vi "preregister_tools.vi"() -> ()   [LabVIEW 2018]
uses:
  controls/preregistration_data.ctl
panel:
  out "text":string
  in  "preregistration_data":T1 {"Starting serial number" format="%#_11g"}
  out "error out":errorcluster
  in  "close":bool
  out "Progress of preregistration data generation":u8(slide) scale=0.0..100.0
  out "Progress of mac_db.txt generation":u8(slide) scale=0.0..100.0
  in  "open":bool
  in  "run":bool
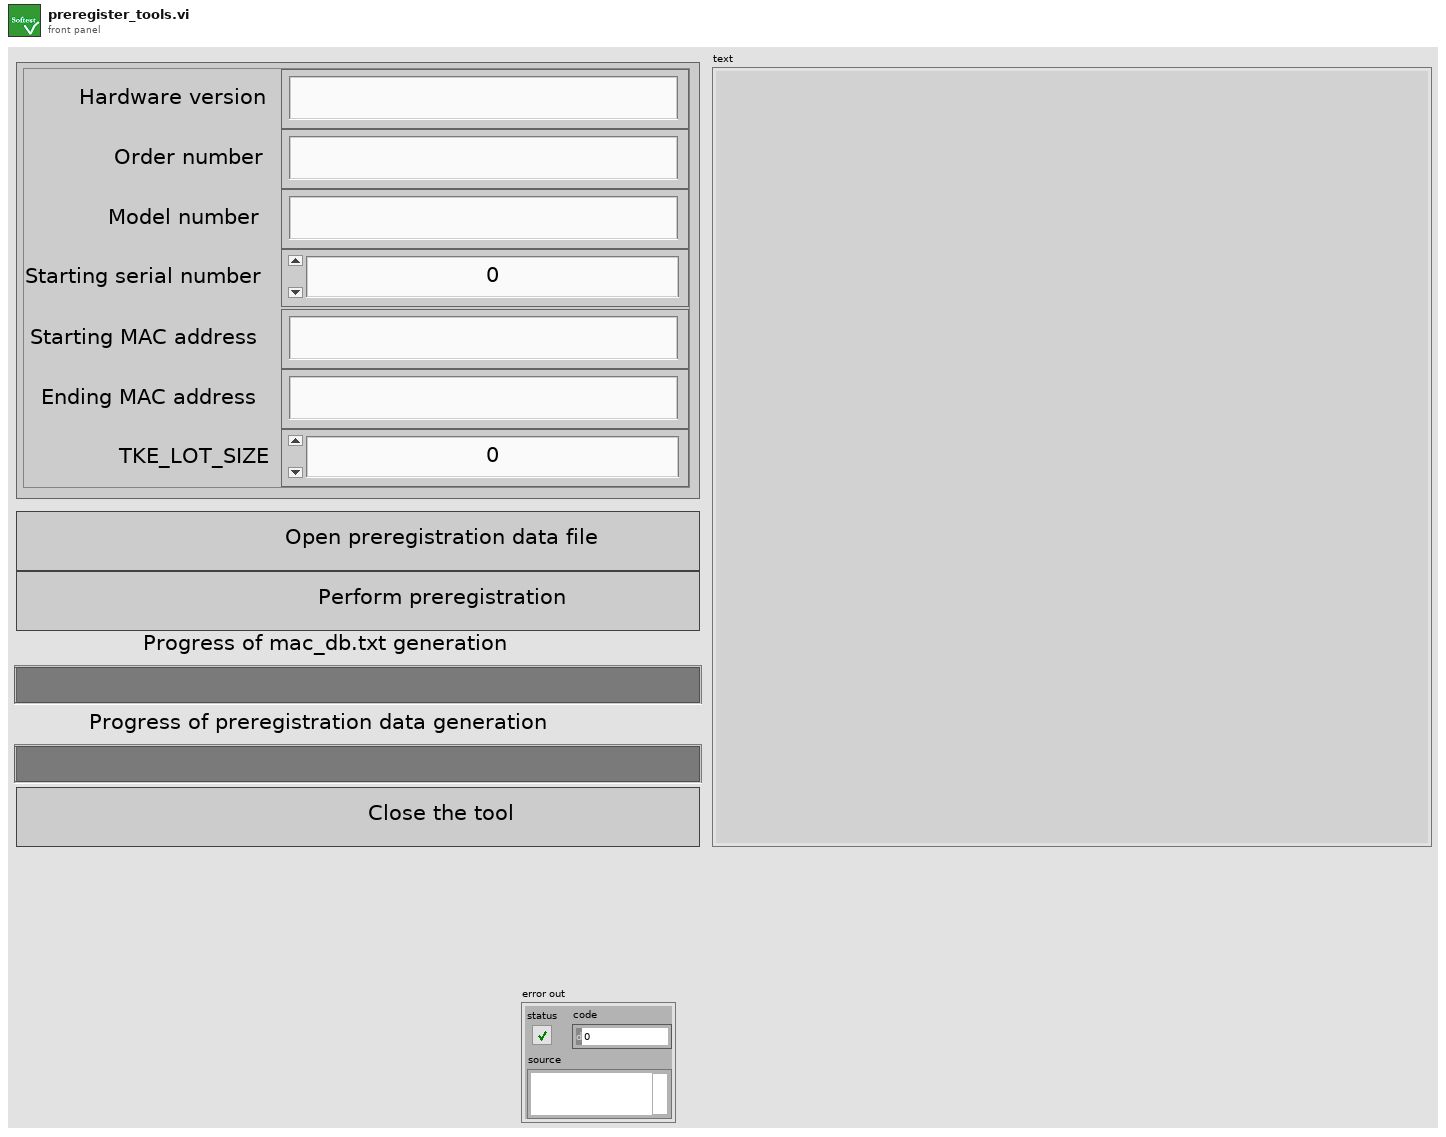
[diagram p1: front panel]
types:
  T1 = typedef "preregistration_data.ctl" = cluster{"Hardware version":string, "Order number":string, "Model number":string, "Starting serial number":i32, "Starting MAC address":string, "Ending MAC address":string, "TKE_LOT_SIZE":i32}
  T2 = enum32{"invalid app kind", "Development System", "Run Time System", "Student Edition", "Embedded LabVIEW", "Evaluation", "Custom"}
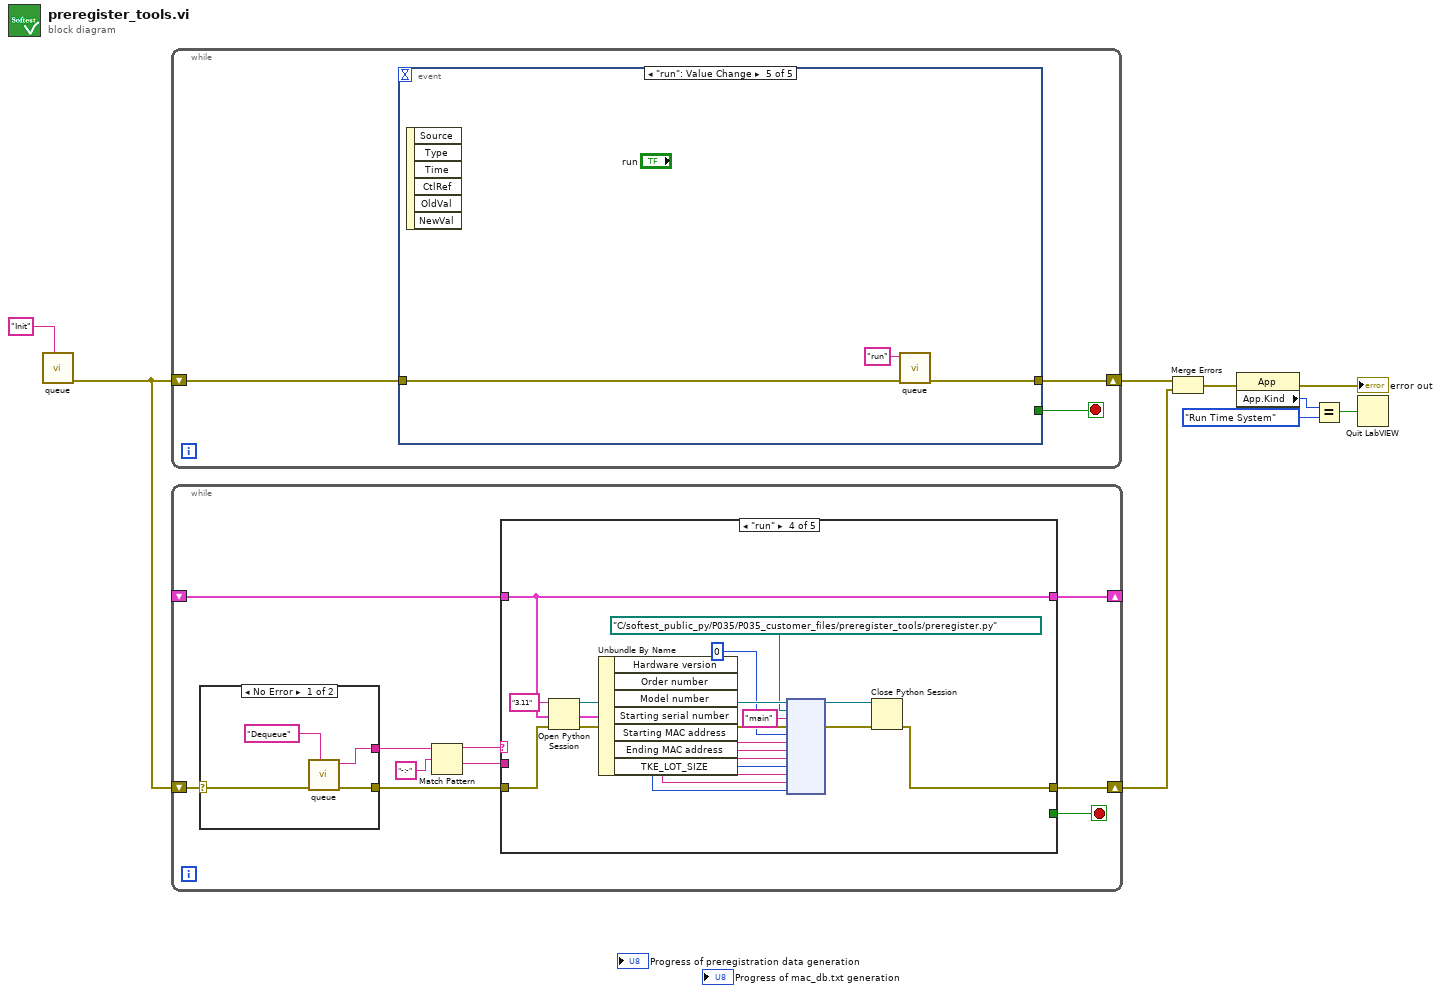
[diagram p0: block diagram]
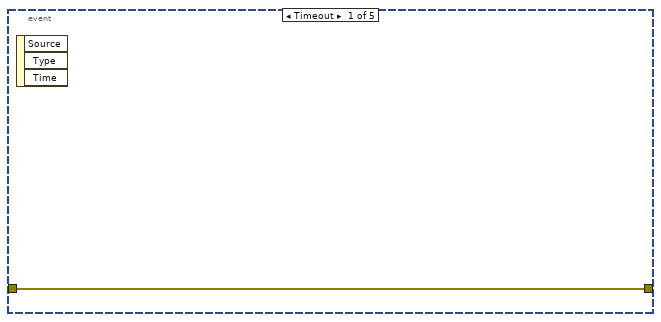
[diagram p2: hidden frame]
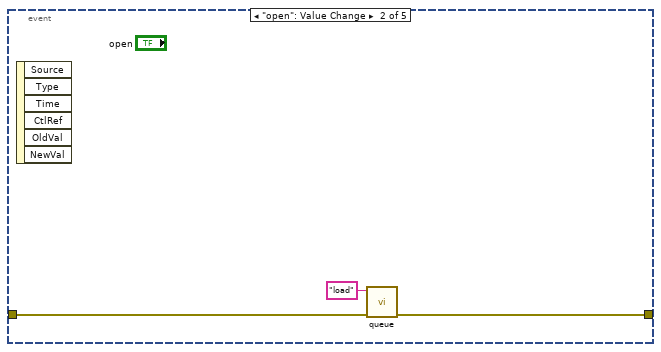
[diagram p3: hidden frame]
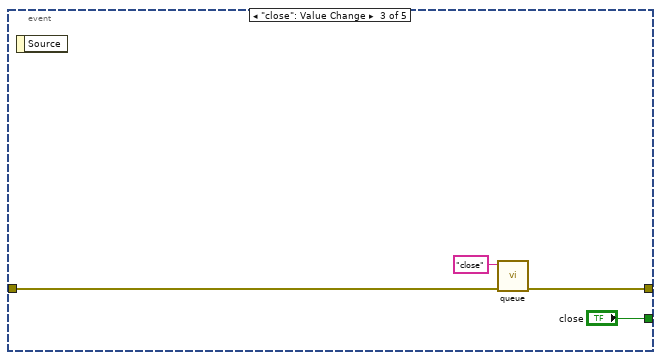
[diagram p4: hidden frame]
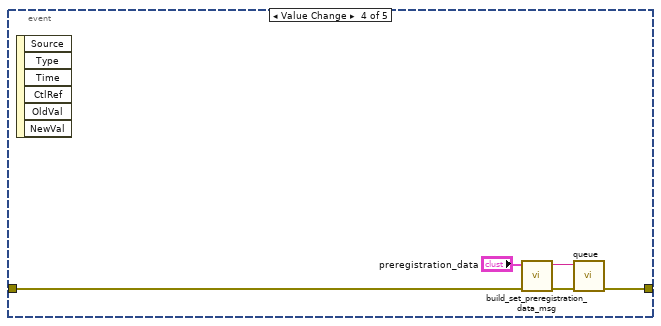
[diagram p5: hidden frame]
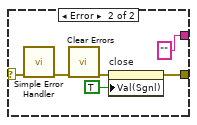
[diagram p6: hidden frame]
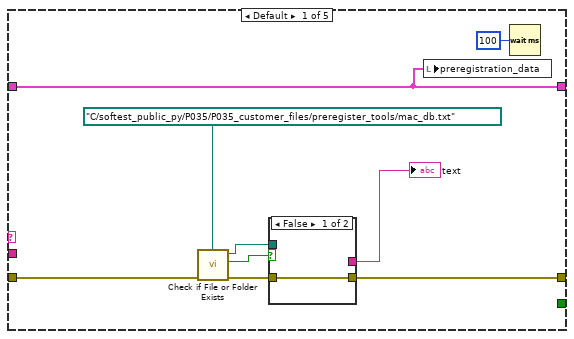
[diagram p7: hidden frame]
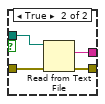
[diagram p8: hidden frame]
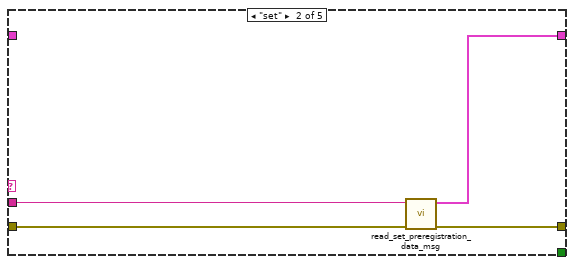
[diagram p9: hidden frame]
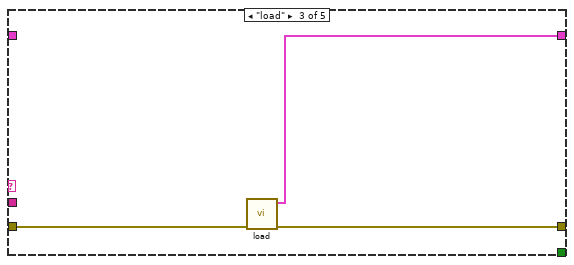
[diagram p10: hidden frame]
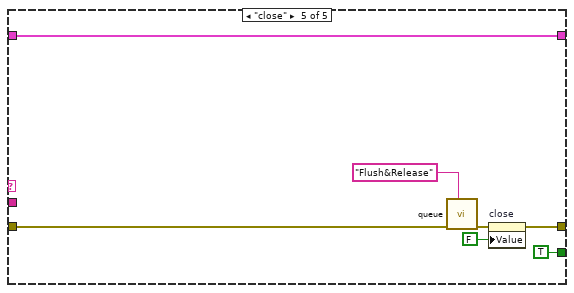
[diagram p11: hidden frame]
diagram:
  n1 = call "queue.vi"("action"="Init") -> ("error_out"=w8:errorcluster)  [unwired: 9 in, 1 out]
  n2 = while {
    shift-right: [w10] -> w7
    shift-left: w8 -> [w11]
    stop <- w12 stop-if-true
    n3 = event shown="[4] \"run\": Value Change" {
      selector: _ -> [_ _ _ _ _]
      dyn-events: _ -> [_ _ _ _ _]
      timeout: _ -> [_ _ _ _ _]
      tunnel: [_ _ "close" _ _] -> w12
      tunnel: w11 -> [w13 w16 w19 w24 w28]
      tunnel: [w13 w15 w18 w25 w27] -> w10
      event Timeout {
        n4 = event-data() -> ()  [unwired: 1 in, 3 out]
      }
      event "open": Value Change {
        n5 = event-data() -> ()  [unwired: 1 in, 6 out]
        n6 = call "queue.vi"("error_in"=w16, "element_in"="load") -> ("error_out"=w15:errorcluster)  [unwired: 8 in, 1 out]
      }
      event "close": Value Change {
        n7 = event-data() -> ()  [unwired: 1 in, 1 out]
        n8 = call "queue.vi"("error_in"=w19, "element_in"="close") -> ("error_out"=w18:errorcluster)  [unwired: 8 in, 1 out]
      }
      event Value Change {
        n9 = event-data() -> ()  [unwired: 1 in, 6 out]
        n10 = call "build_set_preregistration_data_msg.vi"("error_in"=w24, "preregistration_data"="preregistration_data") -> ("error_out"=w23:errorcluster, "command"=w22:string)  [unwired: 8 in]
        n11 = call "queue.vi"("error_in"=w23, "element_in"=w22) -> ("error_out"=w25:errorcluster)  [unwired: 8 in, 1 out]
      }
      event "run": Value Change {
        n12 = event-data() -> ()  [unwired: 1 in, 6 out]
        n13 = call "queue.vi"("error_in"=w28, "element_in"="run") -> ("error_out"=w27:errorcluster)  [unwired: 8 in, 1 out]
      }
    }
  }
  n14 = while {
    shift-right: [w37] -> w6
    shift-left: w8 -> [w35]
    shift-right: [w34] -> _
    shift-left: _ -> [w33]
    stop <- w38 stop-if-true
    n15 = case shown="No Error" w35 {
      selector: w35 -> [w39 w47]
      tunnel: [w42 w44] -> w36
      tunnel: [w41 "" ("element_out")] -> w32
      frame No Error {
        n16 = call "queue.vi"("action"="Dequeue", "error_in"=w39) -> ("error_out"=w42:errorcluster, "element_out"=w41:string)  [unwired: 8 in]
      }
      frame Error {
        n17 = call <vilib>:"Simple Error Handler.vi"("error in (no error)"=w47) -> ("error out"=w46:errorcluster)  [unwired: 4 in, 4 out]
        n18 = call <vilib>:"Clear Errors.vi"("error in (no error)"=w46) -> ("error out"=w45:errorcluster)  [unwired: 5 in, 1 out]
        n19 = property on="close" class="Bool (strict)"(error in=w45, "Val(Sgnl)"=TRUE) -> (error out=w44:errorcluster)  [unwired: 1 in, 1 out]
      }
    }
    n20 = Match Pattern(string=w32, regular expression="-:-") -> (before substring=w30:string, after substring=w29:string)  [unwired: 1 in, 2 out]
    n21 = case shown="\"run\"" w30 {
      tunnel: [_ _ _ _ TRUE] -> w38
      tunnel: w36 -> [w53 w66 w68 w82 w93]
      tunnel: [w54 w64 w69 w83 w90] -> w37
      tunnel: [w56 w63 w67 w79 w88] -> w34
      tunnel: w33 -> [w56 _ _ w79 w88]
      tunnel: w29 -> [_ w65 _ _ _]
      frame Default {
        n22 = call <vilib>:"Check if File or Folder Exists.vi"("error in (no error)"=w53, "path"=path "C:/softest_public_py/P035/P035_customer_files/preregister_tools/mac_db.txt") -> ("error out"=w52:errorcluster, "file or folder exists?"=w51:bool, "dup path"=w50:path)  [unwired: 7 in]
        n23 = case shown="False" w51 {
          tunnel: [_ w62] -> w55
          tunnel: [w58 w61] -> w54
          tunnel: w52 -> [w58 w60]
          tunnel: w50 -> [_ w59]
          frame False {
          }
          frame True {
            n24 = Read from Text File(file (use dialog)=w59, error in=w60) -> (text=w62:string, error out=w61:errorcluster)  [unwired: 2 in, 2 out]
          }
        }
        "text" <- w55
        n25 = local write "preregistration_data"(w56) -> ()
        n26 = Wait (ms)(milliseconds to wait=u32 100) -> ()  [unwired: 1 out]
      }
      frame "set" {
        n27 = call "read_set_preregistration_data_msg.vi"("error_in"=w66, "command"=w65) -> ("error_out"=w64:errorcluster, "preregistration_data"=w63:T1)  [unwired: 8 in]
      }
      frame "load" {
        n28 = call "load.vi"("error in (no error)"=w68) -> ("error out"=w69:errorcluster, "preregistraion_data"=w67:T1)  [unwired: 9 in]
      }
      frame "run" {
        n29 = Open Python Session(python version="3.11" ("Python version"), 3:w82) -> (session out=w87:refnum<k35>, error out=w85:errorcluster)  [unwired: 1 in]
        n30 = Unbundle By Name(w79) -> ("Hardware version"=w77:string, "Order number"=w76:string, "Model number"=w75:string, "Starting serial number"=w74:i32, "Starting MAC address"=w73:string, "Ending MAC address"=w72:string, "TKE_LOT_SIZE"=w71:i32)
        n31 = node(w87, path "C:/softest_public_py/P035/P035_customer_files/preregister_tools/preregister.py" ("module path"), "main" ("function name"), w85, 0, w77, w76, w75, w74, w73, w72, w71) -> (w86:refnum<k35>, w84:errorcluster)  [unwired: 8 in, 2 out]
        n32 = Close Python Session(session in=w86, error in=w84) -> (11:w83:errorcluster)
      }
      frame "close" {
        n33 = call "queue.vi"("action"="Flush&Release", "error_in"=w93) -> ("error_out"=w91:errorcluster)  [unwired: 8 in, 1 out]
        n34 = property on="close" class="Bool (strict)"(error in=w91, "Value"=FALSE ("close")) -> (error out=w90:errorcluster)  [unwired: 1 in, 1 out]
      }
    }
  }
  n35 = Merge Errors(w7, w6) -> (w5:errorcluster)
  n36 = property class="App"(error in=w5) -> (error out=→"error out":errorcluster, "App.Kind"=w3:T2)  [unwired: 1 in, 1 out]
  n37 = Equal?(x=w3, y=T2."Run Time System") -> (x = y?=w1:bool)
  n38 = Quit LabVIEW(quit? (T)=w1) -> ()
